vi "Estimate a.vi"(10 "Gamma":dbl[][](array[numeric]), 11 "Xi":dbl[][][](array[numeric])) -> (3 "Estimated a":dbl[][](array[numeric]))   [LabVIEW 2014, in "HMM.lvlib"]
doc: "Estimates the transition matrix (a) with the input HMM model."
uses:
  HMM.lvlib
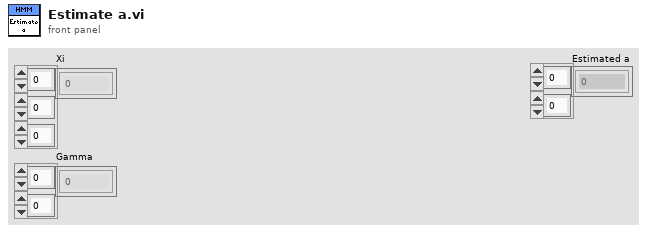
[diagram p1: front panel]
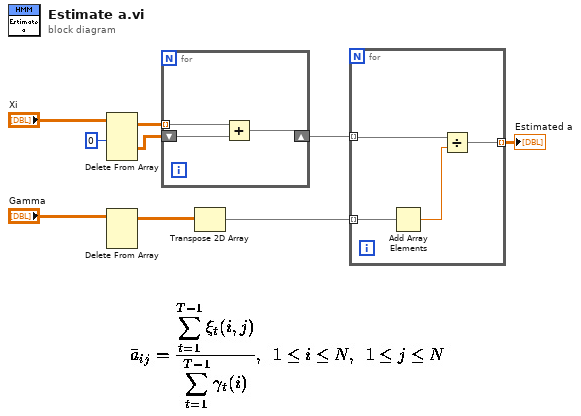
[diagram p0: block diagram]
diagram:
  n1 = Delete From Array(array="Xi", index (dim 0)=0 ("index (page)")) -> (deleted portion=w8:dbl[][], array with subset deleted=w7:dbl[][][])  [unwired: 3 in]
  n2 = Delete From Array(array="Gamma") -> (array with subset deleted=w1:dbl[][])  [unwired: 3 in, 1 out]
  n3 = for {
    tunnel: w7 -> [w12] mode=indexing
    shift-right: [w11] -> w4
    shift-left: w8 -> [w10]
    n4 = Add(x=w12, y=w10) -> (x+y=w11:dbl[][])
  }
  n5 = Transpose 2D Array(2D array=w1) -> (transposed array=w3:dbl[][])
  n6 = for {
    tunnel: w3 -> [w16] mode=indexing
    tunnel: w4 -> [w15] mode=indexing
    tunnel: [w13] -> w6 mode=indexing
    n7 = Add Array Elements(numeric array=w16) -> (sum=w14:dbl)
    n8 = Divide(x=w15, y=w14) -> (x/y=w13:dbl[])
  }
  "Estimated a" <- w6
